vi "DOE Create Capacity String Data.vi"(11 "DOE Capacity Measurments":T1) -> (3 "Capacity Measurement String Output":string[][](array[string]))   [LabVIEW 2016]
uses:
  Type Definitions/DOE Capacity Measurments.ctl
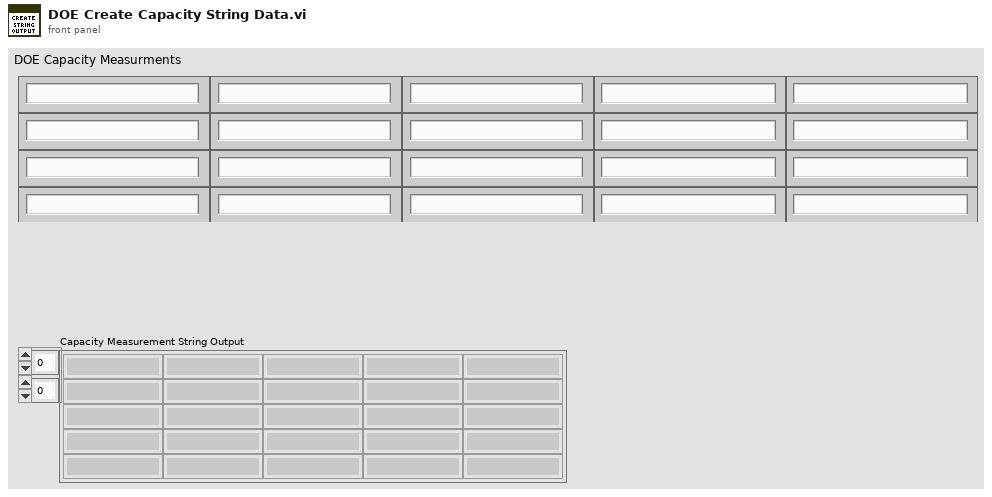
[diagram p1: front panel]
types:
  T1 = typedef "DOE Capacity Measurments.ctl" = cluster{"Weight 1":dbl, "Model Number 1":string, "Temp 1":dbl, "Serial Number 1":string, "Lab Number 1":string, "Lab Number 2":string, "Serial Number 2":string, "Temp 2":dbl, "Model Number 2":string, "Weight 2":dbl, "Lab Number 3":string, "Serial Number 3":string, "Temp 3":dbl, "Model Number 3":string, "Weight 3":dbl, "Lab Number 4":string, "Serial Number 4":string, "Temp 4":dbl, "Model Number 4":string, "Weight 4":dbl, "Capacity Measurment Output String":string[][]}
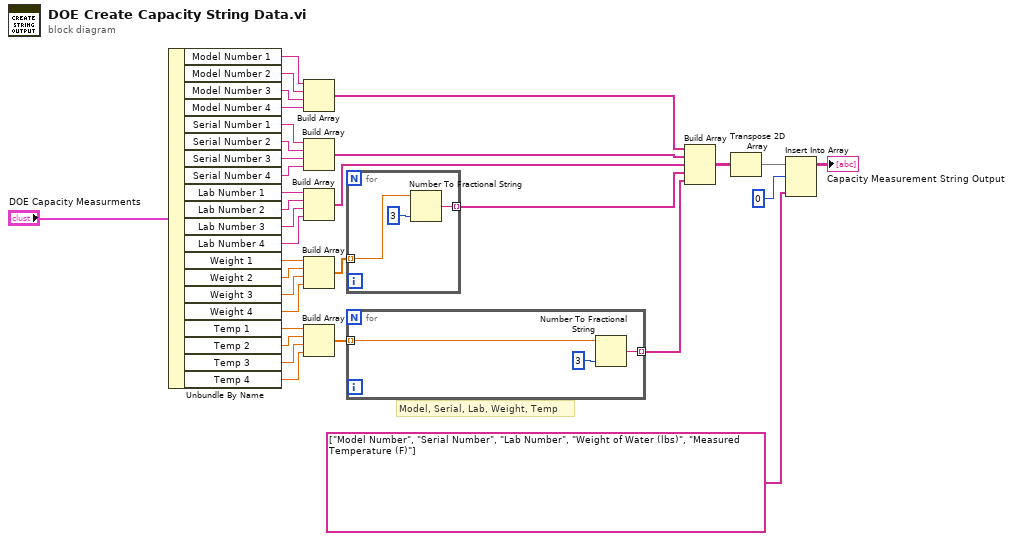
[diagram p0: block diagram]
diagram:
  # "Model, Serial, Lab, Weight, Temp"
  n1 = Unbundle By Name("DOE Capacity Measurments") -> ("Model Number 1"=w12:string, "Model Number 2"=w11:string, "Model Number 3"=w10:string, "Model Number 4"=w9:string, "Serial Number 1"=w26:string, "Serial Number 2"=w25:string, "Serial Number 3"=w24:string, "Serial Number 4"=w23:string, "Lab Number 1"=w22:string, "Lab Number 2"=w21:string, "Lab Number 3"=w20:string, "Lab Number 4"=w19:string, "Weight 1"=w32:dbl, "Weight 2"=w31:dbl, "Weight 3"=w30:dbl, "Weight 4"=w29:dbl, "Temp 1"=w18:dbl, "Temp 2"=w17:dbl, "Temp 3"=w16:dbl, "Temp 4"=w15:dbl)
  n2 = Build Array(w12, w11, w10, w9) -> (w8:string[])
  n3 = Build Array(w26, w25, w24, w23) -> (w7:string[])
  n4 = Build Array(w22, w21, w20, w19) -> (w6:string[])
  n5 = Build Array(w32, w31, w30, w29) -> (w27:dbl[])
  n6 = Build Array(w18, w17, w16, w15) -> (w28:dbl[])
  n7 = for {
    tunnel: w27 -> [w35] mode=indexing
    tunnel: [w34] -> w14 mode=indexing
    n8 = Number To Fractional String(number=w35, precision (6)=i16 3) -> (F-format string=w34:string)  [unwired: 2 in]
  }
  n9 = for {
    tunnel: w28 -> [w39] mode=indexing
    tunnel: [w37] -> w13 mode=indexing
    n10 = Number To Fractional String(number=w39, precision (6)=i16 3) -> (F-format string=w37:string)  [unwired: 2 in]
  }
  n11 = Build Array(w8, w7, w6, w14, w13) -> (w5:string[][])
  n12 = Transpose 2D Array(2D array=w5) -> (transposed array=w4:string[][])
  n13 = Insert Into Array(array=w4, index (row)=0, new element=string[] ["Model Number", "Serial Number", "Lab Number", "Weight of Water (lbs)", "Measured Temperature (F)"]) -> (→"Capacity Measurement String Output":string[][])  [unwired: 1 in]
